vi "Event Self Alias.vi"(11 "jettl in":refnum<class "jettl.lvclass">) -> (2 "Event Self Alias":string)   [LabVIEW 2021, in "jettl.lvlib" / "jettl.lvclass"]
uses:
  jettl.lvclass
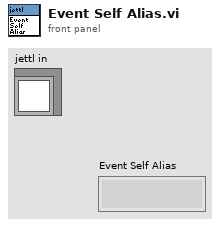
[diagram p1: front panel]
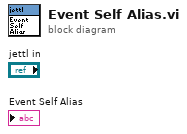
[diagram p0: block diagram]
diagram:
